vi "Bus Interface.vi"(0 "niUSRP DSP v2 FPGA":refnum<class "niUSRP Rx DSP v2 FPGA.lvclass">, 1 "abort":bool, 5 "instruction":T2, 9 "input valid":bool) -> (6 "response":T1, 10 "done":bool, 14 "ready for input":bool)   [LabVIEW 2025, in "niUSRP Rx DSP v2 FPGA.lvclass"]
uses:
  niUSRP Rx DSP v2 FPGA.lvclass
  <instrlib>/_niInstr/Instruction Framework/v1/FPGA/Interfaces/Address Space/Address Space Instruction.ctl
  <instrlib>/_niInstr/Instruction Framework/v1/FPGA/Typedefs/Response.ctl
  niUSRP Rx DSP v2 FPGA.lvclass/niUSRP Rx DSP v2 FPGA.ctl
  <vilib>/rvi/DataTransferAndStorage/Container/Common/niFpgaContainerExecOnDevCompGetState.vi
  <vilib>/rvi/Emulation/niFpgaEmulationIsFPGAContextNoSignature.vi
  <vilib>/rvi/DataTransferAndStorage/Container/Common/niFpgaContainerGetUniqueNameForEmu.vi
  <vilib>/rvi/Memory/Memory_Emulation/niFpgaMemoryEmulationCacheClearOnFirstRun.vi
  <vilib>/rvi/Memory/Memory_Emulation/nirvimemoryEmulationManagerCache_MakeExclusive.vi
  <vilib>/rvi/Memory/Memory_Emulation/niFpgaMemoryEmulationValidateCache.vi
  <vilib>/rvi/Memory/Memory_Emulation/nirvimemoryEmulationManagerCache_InsertValue.vi
  <vilib>/Utility/error.llb/Clear Errors.vi
  <vilib>/rvi/Memory/Memory_Emulation/nirvimemoryEmulationManagerCache_ReleaseExclusive.vi
  <vilib>/rvi/Memory/Memory_Emulation/nirvimemoryEmulationManagerCache_GetValue.vi
  <vilib>/rvi/Memory/Memory_Emulation/nirvimemoryEmulationManagerCache_SetValue.vi
  <vilib>/rvi/Emulation/niFpgaProcessEmulError.vi
  <vilib>/rvi/Emulation/niFpgaSctlEmulationGetInTimedLoop.vi
  <vilib>/rvi/DataTransferAndStorage/Container/XNode/niFpgaContainer.xnode
  <vilib>/rvi/DataTransferAndStorage/Register/Emulation/niFpgaRegisterEmulationRefIn.vi
  <instrlib>/_niInstr/Instruction Framework/v1/FPGA/Typedefs/niInstr Instruction Framework v1 FPGA.lvlib
  <instrlib>/_niInstr/Instruction Framework/v1/FPGA/Interfaces/Address Space/Address Space.lvclass
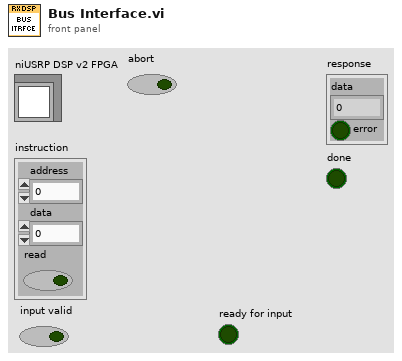
[diagram p1: front panel]
types:
  T1 = typedef "niInstr Instruction Framework v1 FPGA.lvlib/Response.ctl" = cluster{"data":u64, "error":bool}
  T2 = typedef "niInstr Instruction Framework Interfaces v1 FPGA.lvlib/Address Space.lvclass/Address Space Instruction.ctl" = cluster{"address":u32, "data":u64, "read":bool}
  T3 = typedef "niUSRP Rx DSP v2 FPGA.lvclass/DSP Shared Regs.ctl" = cluster{"rfsa.abort":refnum<k21>, "reset":refnum<k21>, "reset.done":refnum<k21>, "RxDspEnabled":refnum<k21>}
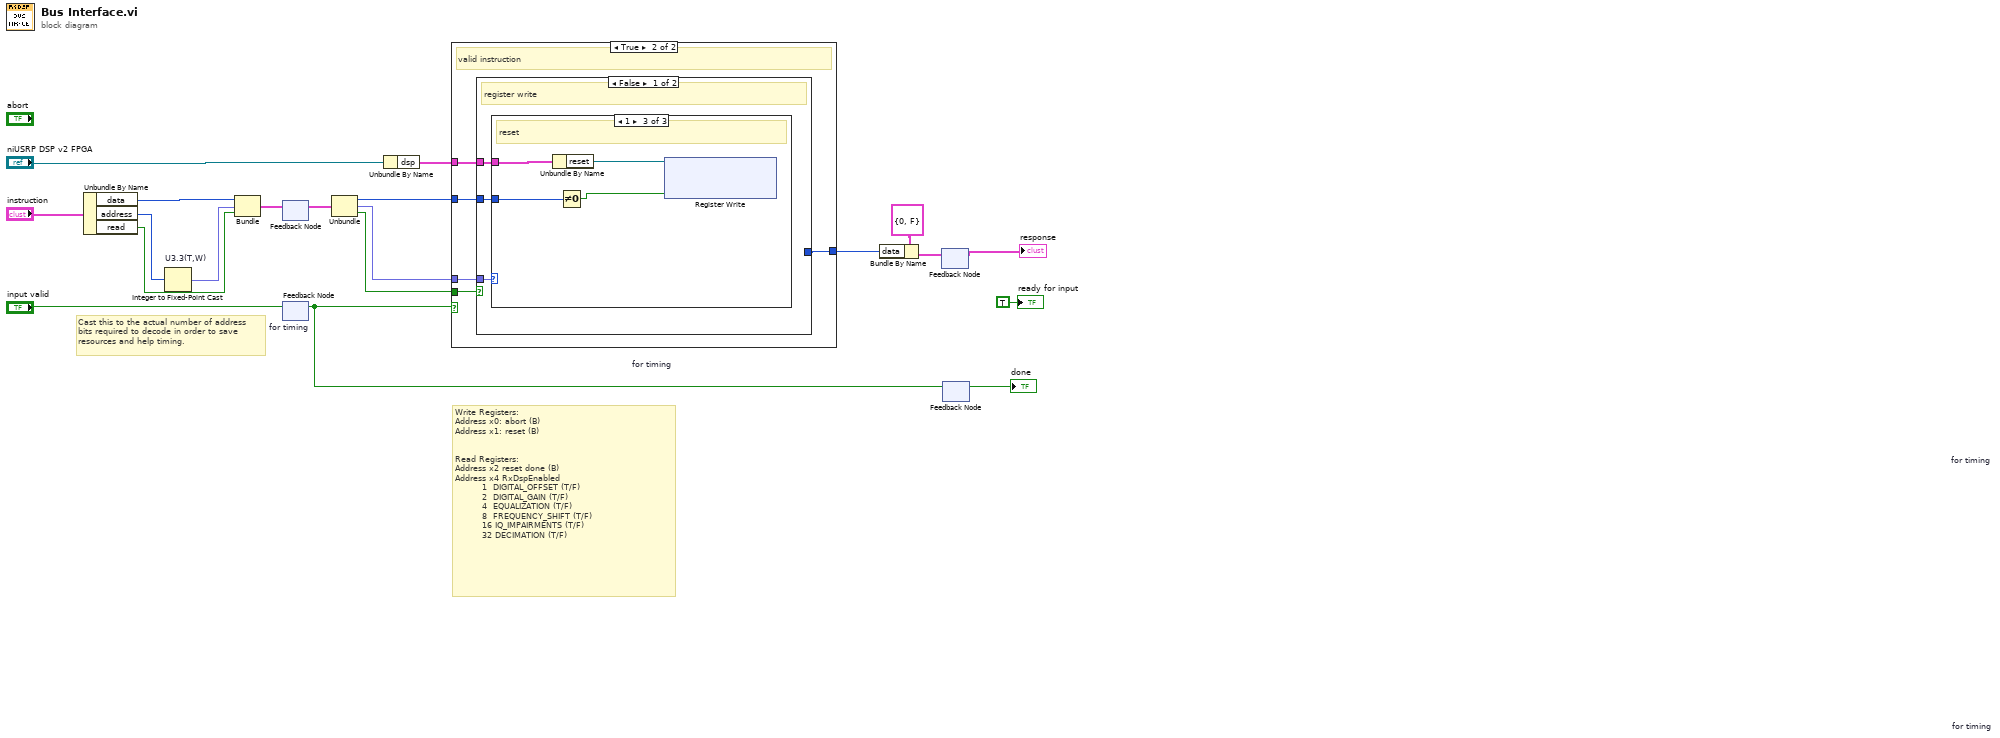
[diagram p0: block diagram]
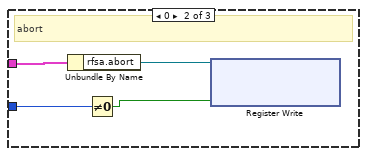
[diagram p4: hidden frame]
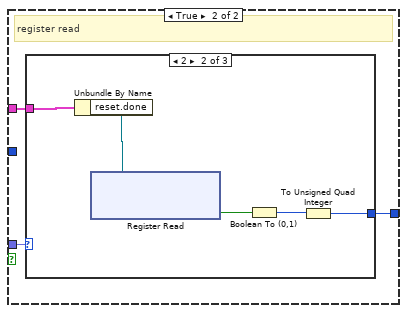
[diagram p5: hidden frame]
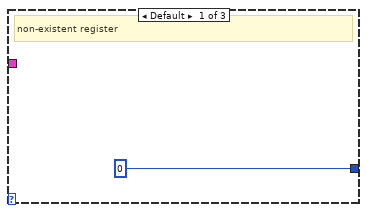
[diagram p6: hidden frame]
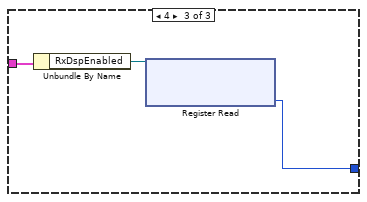
[diagram p7: hidden frame]
diagram:
  # "Write Registers:\nAddress x0: abort (B)\nAddress x1: reset (B)\n\n\nRead Registers:\nAddress x2 reset done (B)\nAddress x4 RxDspEnabled\n         1  DIGITAL_OFFSET (T/F)\n         2  DIGITAL_GAIN (T/F)\n         4  EQUALIZATION (T/F)\n         8  FREQUENCY_SHIFT (T/F)\n         16 IQ_IMPAIRMENTS (T/F)\n         32 DECIMATION (T/F)"
  # "Cast this to the actual number of address\nbits required to decode in order to save\nresources and help timing."
  n1 = Unbundle By Name("instruction") -> ("data"=w17:u64, "address"=w20:u32, "read"=w15:bool)
  n2 = Integer to Fixed-Point Cast "U3.3(T,W)"(integer=w20) -> (fixed-point=w16:fxp<+,3,3>)  [unwired: 1 in]
  n3 = Bundle("data"=w17, w16, "read"=w15) -> (w19:cluster{"data":u64, fxp<+,3,3>, "read":bool})  [unwired: 1 in]
  n4 = feedback #1 "for timing"() -> (w18:cluster{"data":u64, fxp<+,3,3>, "read":bool})  [unwired: 1 in]
  n5 = feedback-in #1(w19) -> ()
  n6 = feedback #2 "for timing"() -> (w7:bool)  [unwired: 1 in]
  n7 = feedback-in #2("input valid") -> ()
  n8 = Unbundle(w18) -> ("data"=w11:u64, w12:fxp<+,3,3>, "read"=w13:bool)
  n9 = Unbundle By Name("niUSRP DSP v2 FPGA") -> ("dsp"=w14:T3)
  n10 = case shown="True" w7 {
    tunnel: w14 -> [_ w25]
    tunnel: w13 -> [_ w24]
    tunnel: w12 -> [_ w23]
    tunnel: w11 -> [_ w22]
    tunnel: [_ w21] -> w10
    frame False {
      # "invalid instruction"
    }
    frame True {
      # "valid instruction"
      n11 = case shown="False" w24 {
        tunnel: w23 -> [w28 w39]
        tunnel: [_ w38] -> w21
        tunnel: w22 -> [w27 _]
        tunnel: w25 -> [w26 w37]
        frame False {
          # "register write"
          n12 = case shown="1" w28 {
            tunnel: w27 -> [_ w30 w34]
            tunnel: w26 -> [_ w31 w35]
            frame Default {
              # "non-existent register"
            }
            frame 0 {
              # "abort"
              n13 = Unbundle By Name(w31) -> ("rfsa.abort"=w32:refnum<k21>)
              n14 = Not Equal To 0?(x=w30) -> (x != 0?=w29:bool)
              n15 = xnode ("Register Write")("Data"=w29, "Register In"=w32) -> ()  [unwired: 1 out]
            }
            frame 1 {
              # "reset"
              n16 = Unbundle By Name(w35) -> ("reset"=w36:refnum<k21>)
              n17 = Not Equal To 0?(x=w34) -> (x != 0?=w33:bool)
              n18 = xnode ("Register Write")("Data"=w33, "Register In"=w36) -> ()  [unwired: 1 out]
            }
          }
        }
        frame True {
          # "register read"
          n19 = case shown="2" w39 {
            tunnel: [u64 0 w45 w46] -> w38
            tunnel: w37 -> [_ w43 w48]
            frame Default {
              # "non-existent register"
            }
            frame 2 {
              n20 = Unbundle By Name(w43) -> ("reset.done"=w44:refnum<k21>)
              n21 = xnode ("Register Read")("Register In"=w44) -> ("Data"=w42:bool)  [unwired: 1 out]
              n22 = Boolean To (0,1)(Boolean=w42) -> (0, 1=w41:i16)
              n23 = To Unsigned Quad Integer(1:w41) -> (0:w45:u64)
            }
            frame 4 {
              n24 = Unbundle By Name(w48) -> ("RxDspEnabled"=w47:refnum<k21>)
              n25 = xnode ("Register Read")("Register In"=w47) -> ("Data"=w46:u64)  [unwired: 1 out]
            }
          }
        }
      }
    }
  }
  n26 = Bundle By Name(cluster=T1 {"data"=0, "error"=FALSE} ("response"), "data"=w10) -> (w8:T1)
  n27 = feedback #3 "for timing"() -> (→"response":T1)  [unwired: 1 in]
  n28 = feedback-in #3(w8) -> ()
  n29 = feedback #4 "for timing"() -> (→"done":bool)  [unwired: 1 in]
  n30 = feedback-in #4(w7) -> ()
  "ready for input" <- TRUE ("ready for input")
